vi "Roc_Curve.vi"(8 "error in (no error)":errorcluster caption="entrée d'erreur (pas d'erreur)", 9 "y_score":string[][](array[string]), 10 "y_true":string[][](array[string]), 11 "roc_curve":T2={"pos_label"={"dtype_pos_label"="None", "pos_label"="None"}, "sample_weight"=[], "drop_intermediate"=TRUE, "Returns"="fpr"}) -> (0 "error out":errorcluster caption="sortie d'erreur", 3 "Data":T1)   [LabVIEW 2020]
doc: "Compute Receiver operating characteristic (ROC)\n\nNote : this implementation is restricted to the binary classification task.\n\n\nParameters : \n\n- y_true : array, shape = [n_samples]\nTrue binary labels. If labels are not either {-1, 1} or {0, 1}, then pos_label should be explicitly given.\n\n- y_score : array, shape = [n_samples]\nTarget scores, can either be probability estimates of the positive class, confidence values, or non-thresholded measure of decisions (as returned by “decision_function” on some classifiers).\n\n- pos_label : int or str, default=None\nThe label of the positive class. When pos_label=None, if y_true is in {-1, 1} or {0, 1}, pos_label is set to 1, otherwise an error will be raised.\n\n- sample_weight : array-like of shape (n_samples,), default=None\nSample weights.\n\n- drop_intermediate : boolean, optional (default=True)\nWhether to drop some suboptimal thresholds which would not appear on a plotted ROC curve. This is useful in order to create lighter ROC curves.\n\nReturns : \n\n- fpr : array, shape = [>2]\nIncreasing false positive rates such that element i is the false positive rate of predictions with score >= thresholds[i].\n\n- tpr : array, shape = [>2]\nIncreasing true positive rates such that element i is the true positive rate of predictions with score >= thresholds[i].\n\n- thresholds : array, shape = [n_thresholds]\nDecreasing thresholds on the decision function used to compute fpr and tpr. thresholds[0] represents no instances being predicted and is arbitrarily set to max(y_score) + 1."
uses:
  Roc_Curve.lvclass
panel:
  out "Roc_Curve.lvclass":refnum<class "Roc_Curve.lvclass">
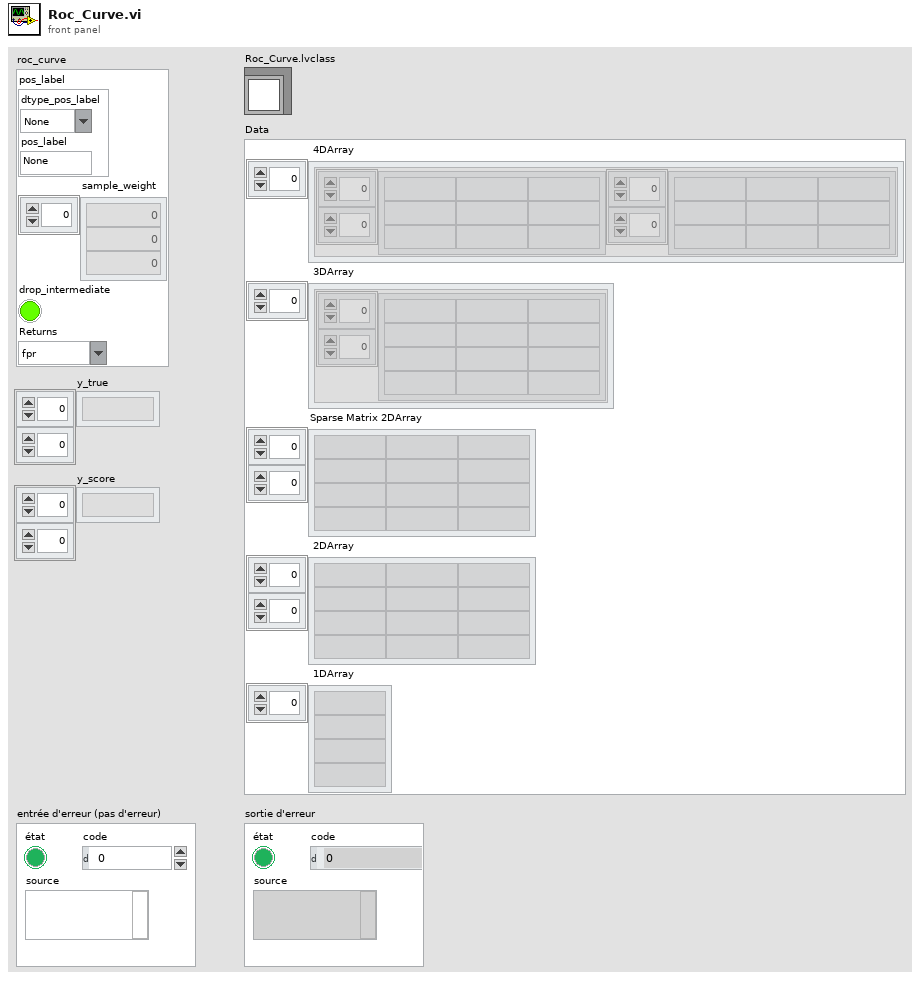
[diagram p1: front panel]
types:
  T1 = cluster{" 4DArray":cluster{"1":string[][], "2":string[][]}[], " 3DArray":cluster{"Tableau":string[][]}[], "Sparse Matrix 2DArray":string[][], " 2DArray":string[][], " 1DArray":string[]}
  T2 = cluster{"pos_label":cluster{"dtype_pos_label":string, "pos_label":string}, "sample_weight":dbl[], "drop_intermediate":bool, "Returns":string}
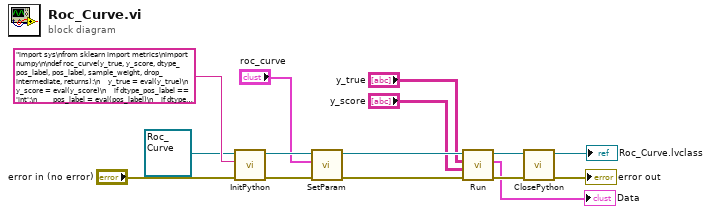
[diagram p0: block diagram]
diagram:
  n1 = call-dynamic "InitPython.vi"("error in (no error)"="error in (no error)", "Python Instruction"="import sys\nfrom sklearn import metrics\nimport numpy\n\ndef roc_curve(y_true, y_score, dtype_pos_label, pos_label, sample_weight, drop_intermediate, returns):\n    y_true = eval(y_true)\n    y_score = eval(y_score)\n    if dtype_pos_label == 'int':\n        pos_label = eval(pos_label)\n    if dtype_pos_label == 'None':\n        pos_label = None\n    if sample_weight == []:\n        sample_weight = None\n    try:\n        fpr, tpr, thresholds = metrics.roc_curve(y_true, y_score, pos_label, sample_weight, drop_intermediate)\n        if returns == 'fpr':\n            roc_curve = fpr.tolist()\n            return str(roc_curve)\n        elif returns == 'tpr':\n            roc_curve = tpr.tolist()\n            return str(roc_curve)\n        else:\n            roc_curve = thresholds.tolist()\n            return str(roc_curve)\n    except:\n        erreur = sys.exc_info()\n        typerr = u\"%s\" % (erreur[0])\n        typerr = typerr[typerr.find(\"'\")+1:typerr.rfind(\"'\")]\n        msgerr = u\"%s\" % (erreur[1])\n        message = str('/!\\\\ {0} : {1}'. format(typerr,msgerr))\n        return message", "Scikit-learn en entrée"=refnum<class "Roc_Curve.lvclass"> refnum ("Roc_Curve.lvclass")) -> ("error out"=w8:errorcluster, "Scikit-learn en sortie"=w10:refnum<class "Roc_Curve.lvclass">)  [unwired: 7 in]
  n2 = call-dynamic "SetParam.vi"("error in (no error)"=w8, "roc_curve"="roc_curve", "Roc_Curve.lvclass"=w10) -> ("error out"=w6:errorcluster, "Roc_Curve.lvclass"=w7:refnum<class "Roc_Curve.lvclass">)  [unwired: 7 in]
  n3 = call-dynamic "Run.vi"("error in (no error)"=w6, "y_score"="y_score", "y_true"="y_true", "Roc_Curve.lvclass"=w7) -> ("error out"=w12:errorcluster, "Data"=→"Data":T1, "Roc_Curve.lvclass"=w11:refnum<class "Roc_Curve.lvclass">)  [unwired: 5 in]
  n4 = call-dynamic "ClosePython.vi"("error in (no error)"=w12, "Scikit-learn en entrée"=w11) -> ("error out"=→"error out":errorcluster, "Scikit-learn en sortie"=→"Roc_Curve.lvclass":refnum<class "Roc_Curve.lvclass">)  [unwired: 8 in]
